vi "Convert MultiSource Variant to Data [DepthFrame].vi"(8 "error in":errorcluster, 11 "MultiSource Variant":variant) -> (0 "error out":errorcluster, 3 "Byte Array":u8[](array[numeric]))   [LabVIEW 2014]
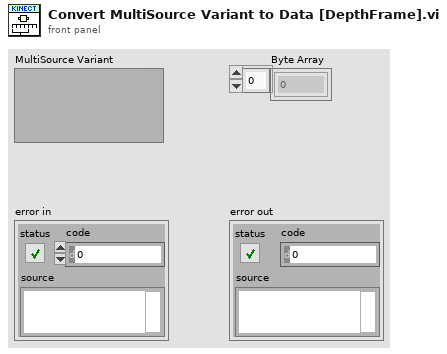
[diagram p1: front panel]
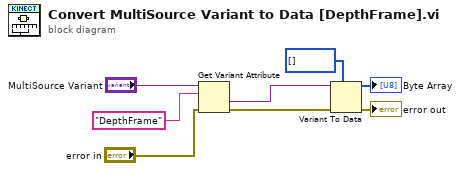
[diagram p0: block diagram]
diagram:
  n1 = Get Variant Attribute(Variant="MultiSource Variant", name="DepthFrame", error in="error in") -> (value=w4:variant, error out=w5:errorcluster)  [unwired: 1 in, 2 out]
  n2 = Variant To Data(error in=w5, type=u8[] [], Variant=w4) -> (data=→"Byte Array":u8[], error out=→"error out":errorcluster)
